vi "AFM_Driver_Manager.SendStop.vi"(8 "error in (no error)":errorcluster, 11 "AFM_Driver_Manager in":refnum<class "AFM_Driver_Manager.lvclass">) -> (0 "error out":errorcluster, 3 "AFM_Driver_Manager out":refnum<class "AFM_Driver_Manager.lvclass">)   [LabVIEW 2020, in "AFM_Driver_Manager.lvclass"]
uses:
  AFM_Driver_Manager.lvclass
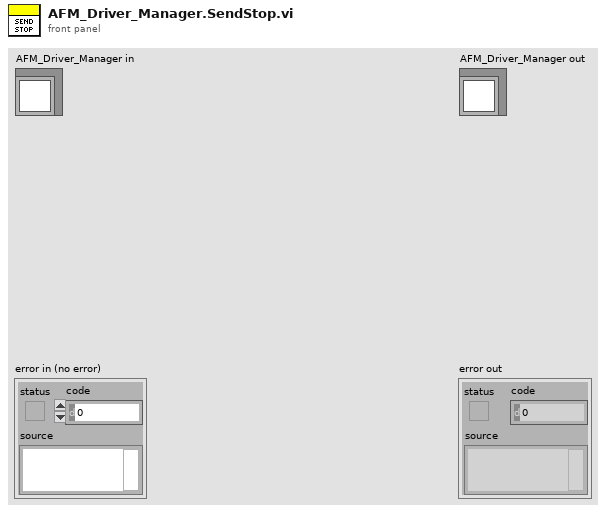
[diagram p1: front panel]
types:
  T1 = typedef "Events.ctl" = cluster{"Stop Event":refnum<user-event>, "Lithography Data":refnum<user-event>, "Run Lithography":refnum<user-event>}
  T2 = cluster{"VI Refnum":refnum<vi>, "Path":path, "Name":string, "Events":T1}
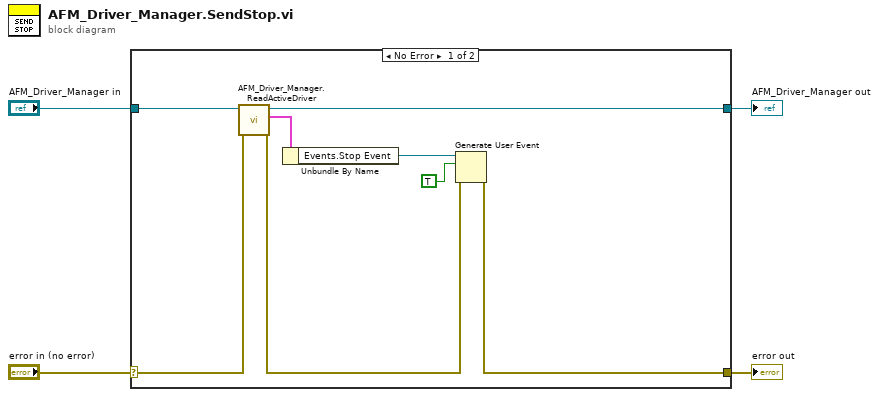
[diagram p0: block diagram]
diagram:
  n1 = case shown="No Error" "error in (no error)" {
    selector: "error in (no error)" -> [w10 w14]
    tunnel: [w5 w14] -> w3
    tunnel: [w12 w13] -> w1
    tunnel: "AFM_Driver_Manager in" -> [w11 w13]
    frame No Error {
      n2 = call "AFM_Driver_Manager.ReadActiveDriver.vi"("error in (no error)"=w10, "AFM_Driver_Manager in"=w11) -> ("error out"=w6:errorcluster, "Active Driver"=w9:T2, "AFM_Driver_Manager out"=w12:refnum<class "AFM_Driver_Manager.lvclass">)  [unwired: 7 in]
      n3 = Unbundle By Name(w9) -> ("Events.Stop Event"=w8:refnum<user-event>)
      n4 = Generate User Event(user event=w8, event data cluster=TRUE ("event data"), error in=w6) -> (error out=w5:errorcluster)  [unwired: 1 in, 1 out]
    }
    frame Error {
    }
  }
  "error out" <- w3
  "AFM_Driver_Manager out" <- w1
